vi "SavePositions3_KCube.vi"(4 "start/stop write":bool, 5 "filename save":string, 6 "init file":bool, 7 "Folder path save":path, 9 "Cluster":T2, 10 "Enum in":T1(ring), 11 "Byte Stream File in":refnum<file>) -> (1 "current state":string, 2 "Enum out":T1(ring), 3 "Byte Stream File out":refnum<file>)   [LabVIEW 2019]
doc: "saves datetime, position value, and isdevicebusy for two dc servo and one channel 1 inertial motor"
uses:
  D:/Victor Sun/optical trap control/Kinesis/ThorLabs.MotionControl.KCube.DCServoCLI.dll
  Kinesis/ThorLabs.MotionControl.KCube.DCServoCLI.dll
  D:/Victor Sun/optical trap control/Kinesis/Thorlabs.MotionControl.KCube.InertialMotorCLI.dll
  Kinesis/Thorlabs.MotionControl.KCube.InertialMotorCLI.dll
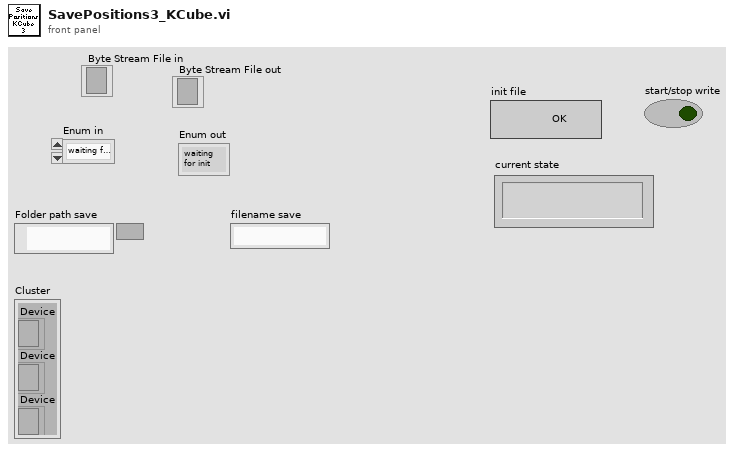
[diagram p1: front panel]
types:
  T1 = enum16{"waiting for init", "init", "waiting for write", "write", "stop", ""}
  T2 = cluster{"Device":refnum<k24>, "Device":refnum<k24>, "Device":refnum<k24>}
  T3 = enum16{"open", "replace", "create", "open or create", "replace or create", "replace or create with confirmation"}
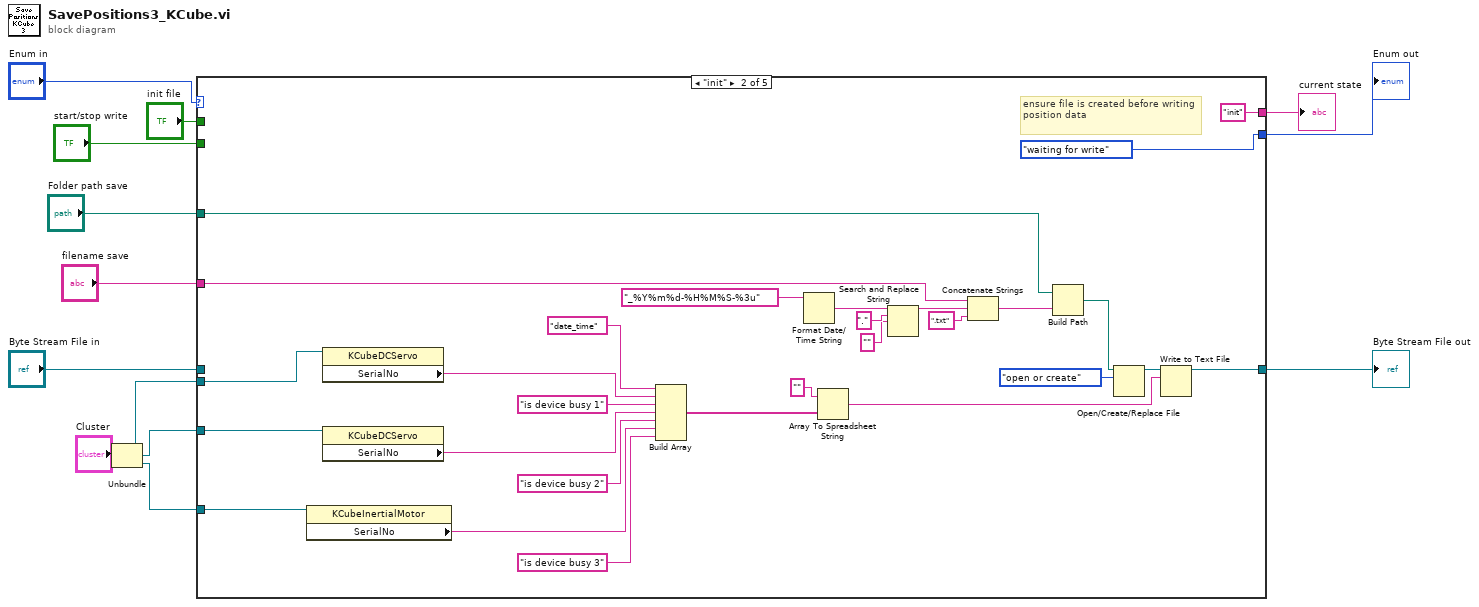
[diagram p0: block diagram]
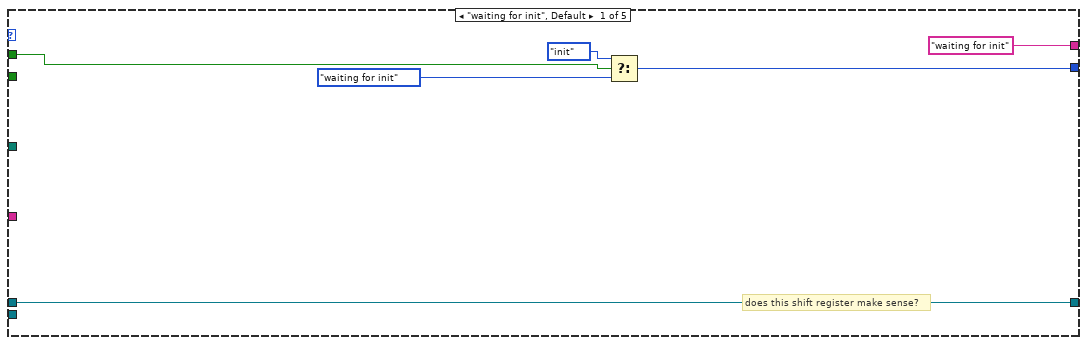
[diagram p2: hidden frame]
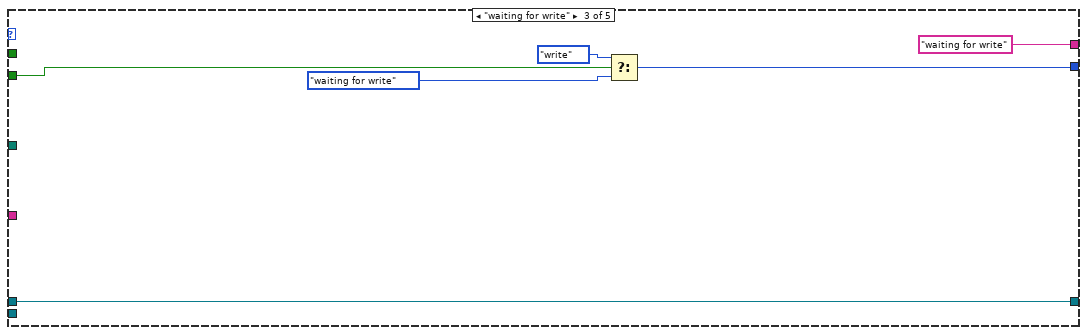
[diagram p3: hidden frame]
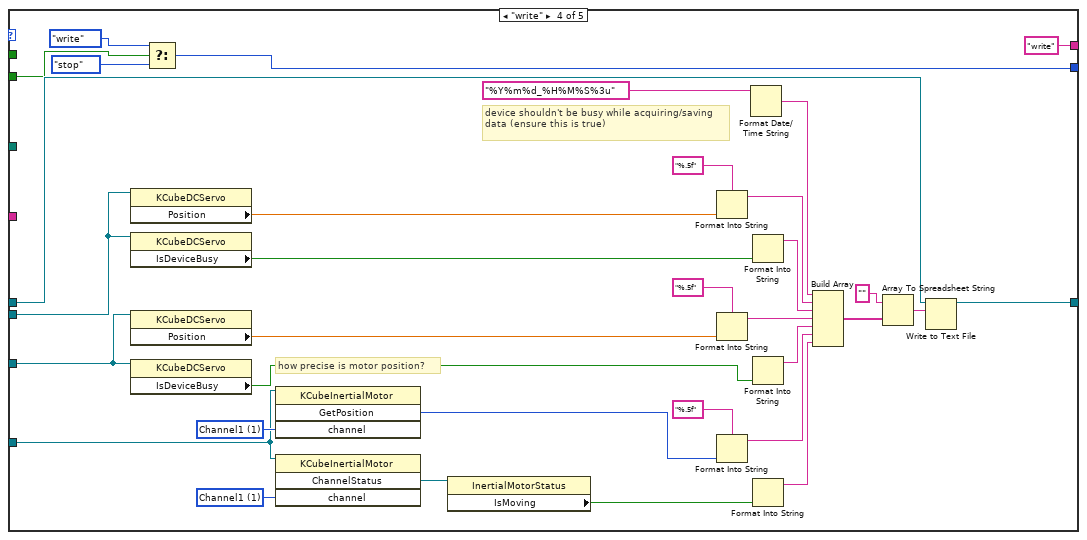
[diagram p4: hidden frame]
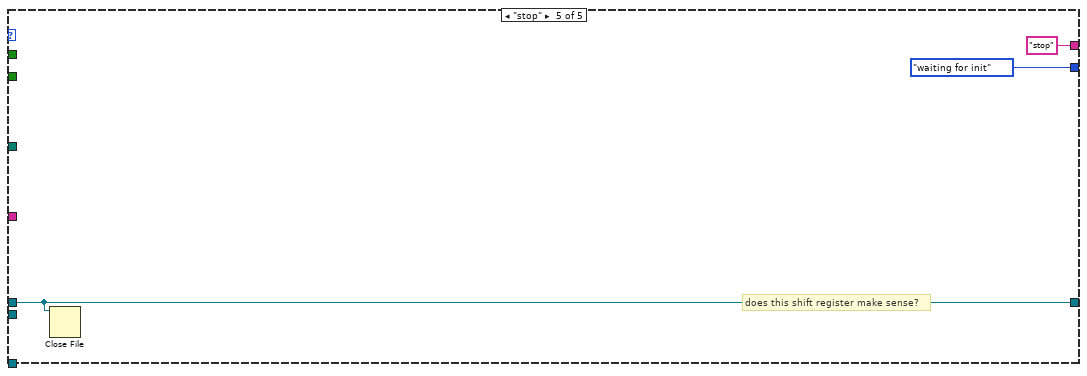
[diagram p5: hidden frame]
diagram:
  n1 = Unbundle("Cluster") -> ("Device"=w12:refnum<k24>, "Device"=w11:refnum<k24>, "Device"=w13:refnum<k24>)
  n2 = case shown="\"init\"" "Enum in" {
    tunnel: [w18 T1."waiting for write" w52 w85 T1."waiting for init"] -> w9
    tunnel: ["waiting for init" ("String") "init" ("String") "waiting for write" ("String") "write" ("String") "stop" ("String")] -> w1
    tunnel: w12 -> [_ w29 _ w83 _]
    tunnel: [w14 w28 w49 w82 w87] -> w2
    tunnel: "Byte Stream File in" -> [w14 _ w49 w84 w87]
    tunnel: "start/stop write" -> [_ _ w48 w71 _]
    tunnel: "init file" -> [w16 _ _ _ _]
    tunnel: "filename save" -> [_ w41 _ _ _]
    tunnel: "Folder path save" -> [_ w38 _ _ _]
    tunnel: w11 -> [_ w25 _ w67 _]
    tunnel: w13 -> [_ w22 _ w66 _]
    frame "waiting for init", Default {
      # "does this shift register make sense?"
      n3 = Select(t=T1."init", s=w16, f=T1."waiting for init") -> (s? t:f=w18:T1)
    }
    frame "init" {
      # "ensure file is created before writing position data"
      n4 = property class="KCubeInertialMotor"(reference=w22) -> ("SerialNo"=w21:string)  [unwired: 1 in, 2 out]
      n5 = property class="KCubeDCServo"(reference=w29) -> ("SerialNo"=w31:string)  [unwired: 1 in, 2 out]
      n6 = property class="KCubeDCServo"(reference=w25) -> ("SerialNo"=w24:string)  [unwired: 1 in, 2 out]
      n7 = Build Array("date_time", w31, "is device busy 1" ("element"), w24, "is device busy 2" ("element"), w21, "is device busy 3" ("element")) -> (w30:string[])
      n8 = Format Date/Time String(time format string (%c)="_%Y%m%d-%H%M%S-%3u") -> (date/time string=w39:string)  [unwired: 2 in]
      n9 = Array To Spreadsheet String(array=w30, 3:"" ("format string")) -> (spreadsheet string=w44:string)  [unwired: 1 in]
      n10 = Search and Replace String(input string=w39, search string=".", replace string="" ("replace string (\"\")")) -> (result string=w40:string)  [unwired: 5 in, 3 out]
      n11 = Concatenate Strings(w41, w40, ".txt" ("result string")) -> (w42:string)
      n12 = Build Path(base path=w38, name or relative path=w42) -> (appended path=w43:path)
      n13 = Open/Create/Replace File(file path (use dialog)=w43, operation (0:open)=T3."open or create") -> (refnum out=w45:refnum<file>)  [unwired: 4 in, 2 out]
      n14 = Write to Text File(file (use dialog)=w45, text=w44) -> (refnum out=w28:refnum<file>)  [unwired: 2 in, 2 out]
    }
    frame "waiting for write" {
      n15 = Select(t=T1."write", s=w48, f=T1."waiting for write") -> (s? t:f=w52:T1)
    }
    frame "write" {
      w65 = 1 items=["Channel1"=1, "Channel2"=2, "Channel3"=3, "Channel4"=4] ("channel")
      w68 = 1 items=["Channel1"=1, "Channel2"=2, "Channel3"=3, "Channel4"=4] ("channel")
      # "device shouldn't be busy while acquiring/saving data (ensure this is true)"
      # "how precise is motor position?"
      n16 = property class="KCubeDCServo"(reference=w83) -> ("Position"=w80:dbl)  [unwired: 1 in, 2 out]
      n17 = property class="KCubeDCServo"(reference=w83) -> ("IsDeviceBusy"=w73:bool)  [unwired: 1 in, 2 out]
      n18 = property class="KCubeDCServo"(reference=w67) -> ("Position"=w55:dbl)  [unwired: 1 in, 2 out]
      n19 = property class="KCubeDCServo"(reference=w67) -> ("IsDeviceBusy"=w61:bool)  [unwired: 1 in, 2 out]
      n20 = Select(t=T1."write", s=w71, f=T1."stop") -> (s? t:f=w85:T1)
      n21 = invoke class="KCubeInertialMotor" method="GetPosition"(reference=w66, "channel"=w68) -> ("GetPosition"=w58:i32)  [unwired: 2 in, 3 out]
      n22 = invoke class="KCubeInertialMotor" method="ChannelStatus"(reference=w66, "channel"=w65) -> ("ChannelStatus"=w63:refnum<k24>)  [unwired: 2 in, 3 out]
      n23 = property class="InertialMotorStatus"(reference=w63) -> ("IsMoving"=w64:bool)  [unwired: 1 in, 2 out]
      n24 = Format Into String(format string="%.5f", w80) -> (resulting string=w77:string)  [unwired: 2 in, 1 out]
      n25 = Format Into String(format string="%.5f", w55) -> (resulting string=w54:string)  [unwired: 2 in, 1 out]
      n26 = Format Into String(format string="%.5f", w58) -> (resulting string=w57:string)  [unwired: 2 in, 1 out]
      n27 = Format Date/Time String(time format string (%c)="%Y%m%d_%H%M%S%3u") -> (date/time string=w78:string)  [unwired: 2 in]
      n28 = Format Into String(w73) -> (resulting string=w72:string)  [unwired: 3 in, 1 out]
      n29 = Format Into String(w61) -> (resulting string=w60:string)  [unwired: 3 in, 1 out]
      n30 = Format Into String(w64) -> (resulting string=w62:string)  [unwired: 3 in, 1 out]
      n31 = Build Array(w78, w77, w72, w54, w60, w57, w62) -> (w76:string[])
      n32 = Array To Spreadsheet String(array=w76, 3:"" ("format string")) -> (spreadsheet string=w75:string)  [unwired: 1 in]
      n33 = Write to Text File(file (use dialog)=w84, text=w75) -> (refnum out=w82:refnum<file>)  [unwired: 2 in, 2 out]
    }
    frame "stop" {
      # "does this shift register make sense?"
      n34 = Close File(refnum=w87) -> ()  [unwired: 1 in, 2 out]
    }
  }
  "current state" <- w1
  "Enum out" <- w9
  "Byte Stream File out" <- w2
